vi "Write Error.vi"(8 "error in (no error)":errorcluster, 10 "error":errorcluster, 11 "AssertEqualValue in":refnum<class "AssertError.lvclass">) -> (0 "error out":errorcluster, 3 "AssertEqualValue out":refnum<class "AssertError.lvclass">)   [LabVIEW 2021, in "Bananas.lvlib" / "AssertError.lvclass"]
uses:
  AssertError.lvclass
  AssertError.lvclass/AssertError.ctl
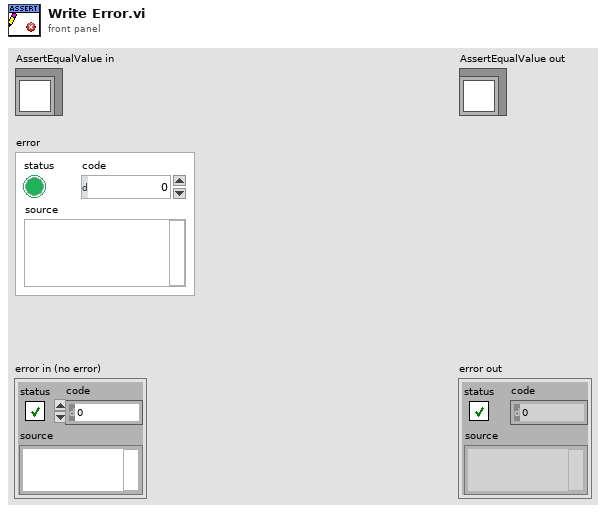
[diagram p1: front panel]
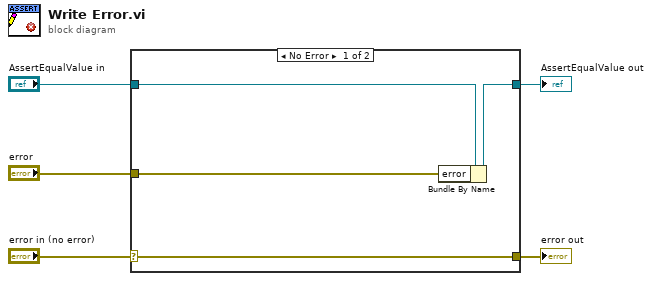
[diagram p0: block diagram]
diagram:
  n1 = case shown="No Error" "error in (no error)" {
    selector: "error in (no error)" -> [w9 w10]
    tunnel: [w9 w10] -> w4
    tunnel: [w6 w11] -> w2
    tunnel: "AssertEqualValue in" -> [w8 w11]
    tunnel: "error" -> [w7 _]
    frame No Error {
      n2 = Bundle By Name(cluster=w8, "error"=w7) -> (w6:refnum<class "AssertError.lvclass">)
    }
    frame Error {
    }
  }
  "error out" <- w4
  "AssertEqualValue out" <- w2
